vi "Read ALRPinitialised.vi"(8 "error in (no error)":errorcluster, 11 "ALR in":T1) -> (0 "error out":errorcluster, 2 "initialised":u8, 3 "ALR out":T1)   [LabVIEW 2019, in "Alarms.lvlib"]
uses:
  Alarms.lvlib
  Ctl/Alarms.ctl
  Ctl/ALR_defs.ctl
  Ctl/ALRs_State.ctl
  Ctl/ALR_ON_OFF.ctl
  Ctl/ALR_Parameters.ctl
  Ctl/ALR code.ctl
  Ctl/ALR type.ctl
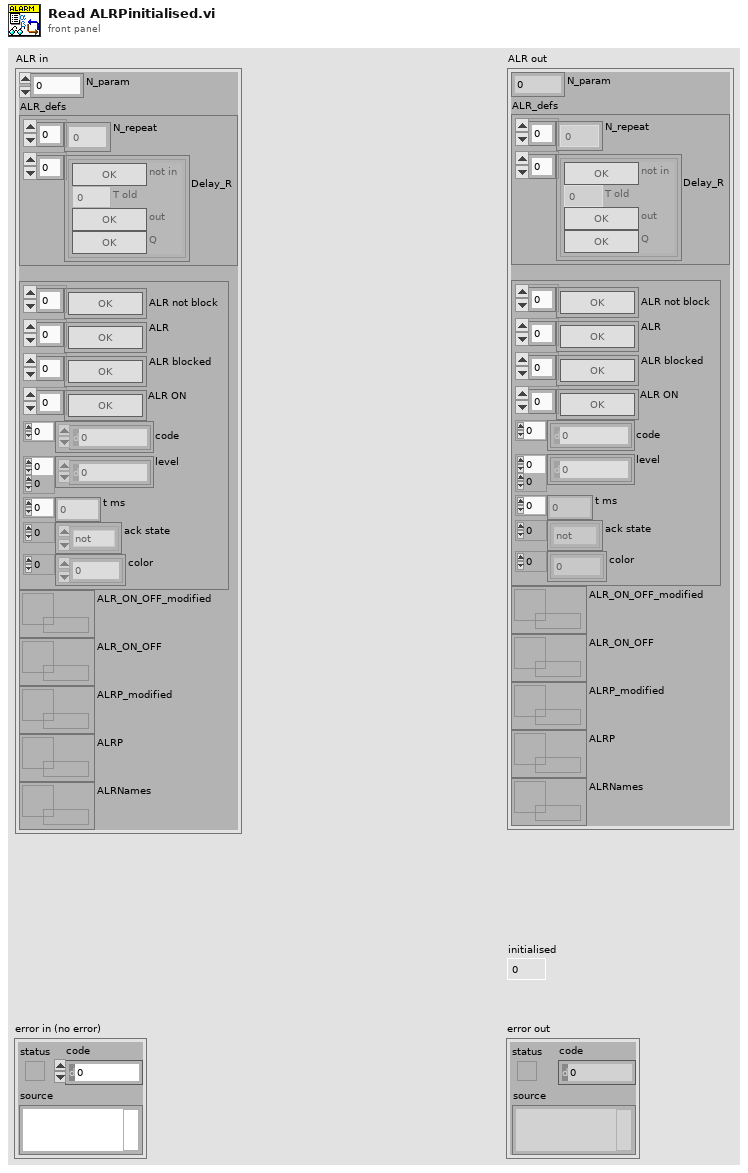
[diagram p1: front panel]
types:
  T1 = typedef "Alarms.lvlib/Alarms.ctl" = cluster{"N_param":i32, "ALR_defs":T2, "ALR_State":T3, "ALR_ON_OFF_modified":refnum<data-value>, "ALR_ON_OFF":refnum<data-value>, "ALRP_modified":refnum<data-value>, "ALRP":refnum<data-value>, "ALRNames":refnum<data-value>}
  T2 = typedef "Alarms.lvlib/ALR_defs.ctl" = cluster{"N_repeat":u32[], "Delay_R":cluster{"not in":bool, "T old":u32, "out":bool, "Q":bool}[]}
  T3 = typedef "Alarms.lvlib/ALRs_State.ctl" = cluster{"ALR not block":bool[], "ALR":bool[], "ALR blocked":bool[], "ALR ON":bool[], "code":i32[], "level":i32[][], "t ms":u32[], "ack state":enum32{"not", "tripped", "reset", "ack"}[], "color":u32[]}
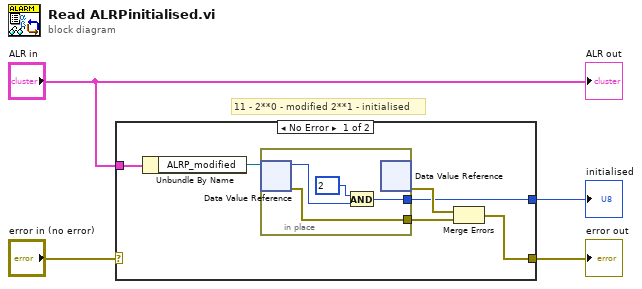
[diagram p0: block diagram]
diagram:
  # "11 - 2**0 - modified 2**1 - initialised"
  n1 = case shown="No Error" "error in (no error)" {
    selector: "error in (no error)" -> [_ w15]
    tunnel: [w10 w15] -> w1
    tunnel: "ALR in" -> [w9 _]
    tunnel: [w6 _] -> w2
    frame No Error {
      n2 = Unbundle By Name(w9) -> ("ALRP_modified"=w8:refnum<data-value>)
      n3 = in-place {
        in-place-border: [w14] -> w5
        in-place-border: [w11] -> w6
        n4 = in-place-dvr #1(w8) -> (w13:u8, w14:errorcluster)
        n5 = And(x=u8 2 ("modified (0)"), y=w13) -> (x .and. y?=w11:u8)
        n6 = in-place-dvr #1() -> (w7:errorcluster)  [unwired: 1 in, 1 out]
      }
      n7 = Merge Errors(w7, w5) -> (w10:errorcluster)
    }
    frame Error {
    }
  }
  "error out" <- w1
  "initialised" <- w2
  "ALR out" <- "ALR in"
